vi "cs-scanning_v4.vi"() -> ()   [LabVIEW 2017]
uses:
  controls/boolean_info.ctl
  controls/TF-params.ctl
  controls/z-axis-params_v4.ctl
  <vilib>/rvi/Emulation/niFpgaGetClockAttributes.vi
  <vilib>/rvi/Emulation/niFpgaSctlEmulationGetInTimedLoop.vi
  <vilib>/rvi/Emulation/niFpgaEmulationReportErrorSimple.vi
  <vilib>/rvi/Emulation/niFpgaProcessEmulError.vi
  <vilib>/rvi/eio/common/nirviEmuTemplateMethod_errors.vi
  <vilib>/rvi/Emulation/niFpgaEmulationIsFPGAContextNoSignature.vi
  <vilib>/rvi/DataTransferAndStorage/Container/Common/niFpgaContainerGetUniqueNameForEmu.vi
  <vilib>/rvi/Memory/Memory_Emulation/niFpgaMemoryEmulationCacheClearOnFirstRun.vi
  <vilib>/rvi/Memory/Memory_Emulation/nirvimemoryEmulationManagerCache_MakeExclusive.vi
  <vilib>/rvi/Memory/Memory_Emulation/niFpgaMemoryEmulationValidateCache.vi
  <vilib>/rvi/Memory/Memory_Emulation/nirvimemoryEmulationManagerCache_InsertValue.vi
  <vilib>/Utility/error.llb/Clear Errors.vi
  <vilib>/rvi/Memory/Memory_Emulation/nirvimemoryEmulationManagerCache_ReleaseExclusive.vi
  <vilib>/rvi/Memory/Memory_Emulation/nirvimemoryEmulationManagerCache_GetValue.vi
  <vilib>/rvi/Memory/Memory_Emulation/nirvimemoryEmulationManagerCache_SetValue.vi
  <vilib>/rvi/Emulation/niFpgaCriticalErrorInLSC.vi
  <vilib>/eio/EIONode/EIONode.xnode
  <vilib>/rvi/DataTransferAndStorage/Container/XNode/niFpgaContainer.xnode
  <vilib>/rvi/DataTransferAndStorage/Register/Emulation/niFpgaRegisterEmulation.vi
  FPGA-data-logging.lvlib
  libimaging-cs.lvlib
panel:
  in  "z_axis_params":T1={"TOL"=0.3, "z_u_max"=5.0, "setpoint-scan"=0.0, "Ki-scan"=0.001, "Z_error_threshold"=0.0, "Z_settled_samples_threshold "=0, "uz_safe"=0.0, "Kiz_down"=0.001, "max_Z_settle_samples"=5000, "setpoint-up"=0.0} {"uz_safe" format="%#_13g"; "Z_error_threshold" format="%#_13g"; "TOL" format="%#_13g"}
  in  "TF-params":T2={"TF-order"=0, "Num"=[0.0, 0.0, 0.0, 0.0, 0.0, 0.0, 0.0, 0.0, 0.0], "Den"=[0.0, 0.0, 0.0, 0.0, 0.0, 0.0, 0.0, 0.0, 0.0]}
  in  "do-Dz":bool
  out "stop_loops":bool
  out "xy_k":fxp<+/-,16,5>[](array[numeric])
  out "xy_ref":fxp<+/-,16,5>[](array[numeric])
  out "u_x saturated":bool
  out "u_y saturated":bool
  out "state1-count":u64
  out "state5-count":u64
  out "state4-count":u64
  out "state3-count":u64
  out "state2-count":u64
  in  "collect all":bool
  out "entity-index":i16
  in  "TsTicks":u32=1600
  out "number-settled-samples-Z":i16
  out "Current Case":u8
  out "boolean \nindicators":T3
  out "z-u(k)":sgl
  in  "ABORT":bool
  out "read fifo timeout":bool
  in  "numEntities":i16
  in  "trigger-0":bool
  out "number-settled-samples-y":i16
  out "number-settled-samples-x":i16
  in  "xy-error-threshold":sgl format="%#_13g"
  in  "settled-samples\nthreshold":i16
  in  "Ki-xy":sgl=0.001 format="%#_13g"
  in  "xy-bound":sgl
  # "- If collect all = fasle ,\nwe only collect measurement data.\n- If collect all = true, we collect everything."
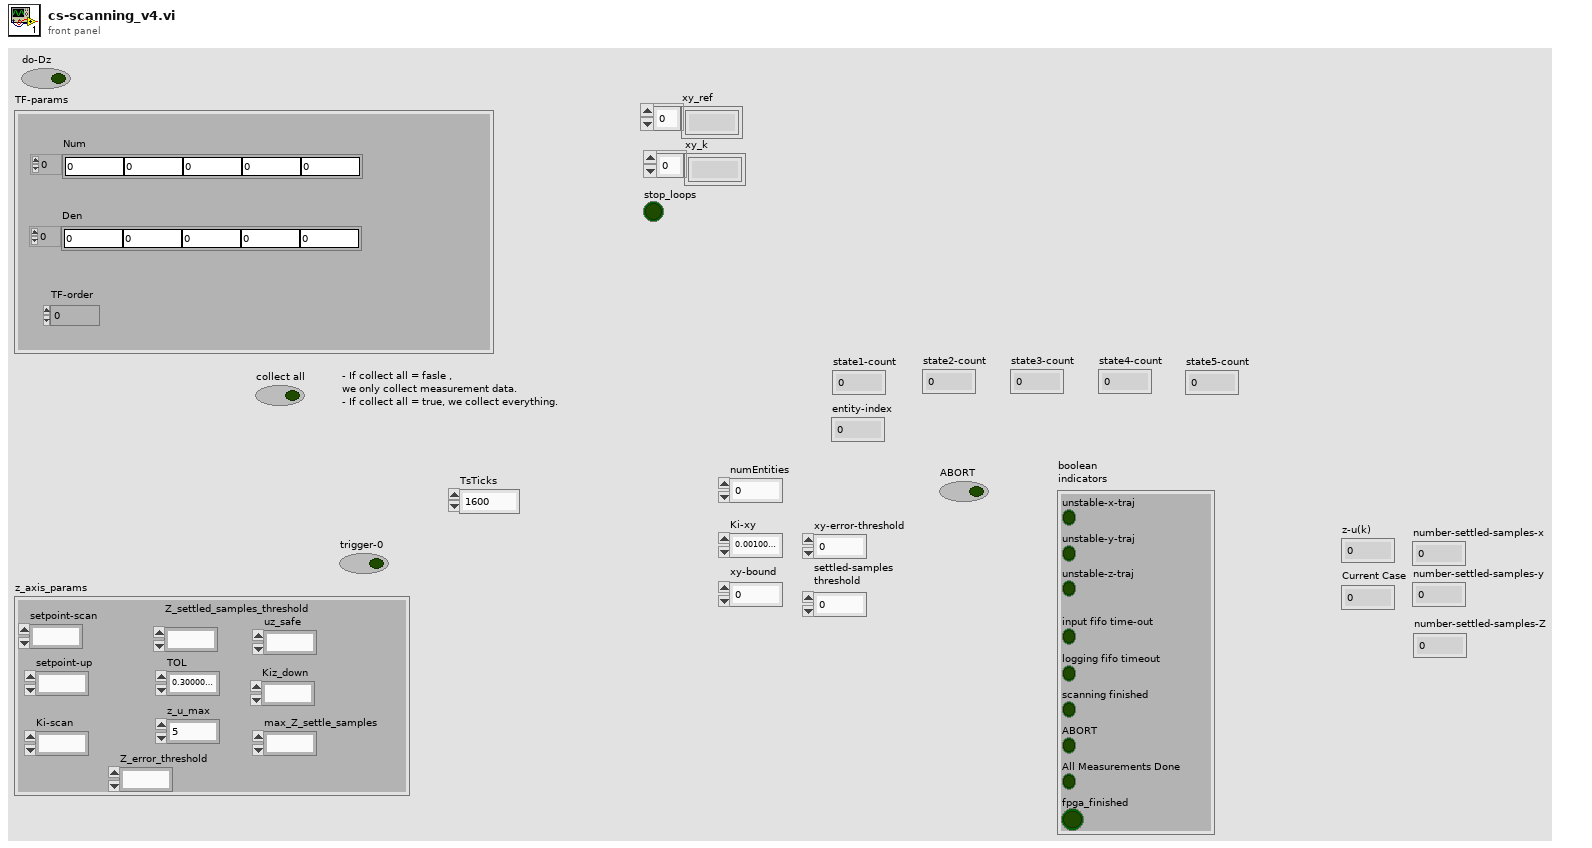
[diagram p1: front panel]
types:
  T1 = typedef "z-axis-params_v4.ctl" = cluster{"TOL":sgl, "z_u_max":sgl, "setpoint-scan":fxp<+/-,32,16>, "Ki-scan":sgl, "Z_error_threshold":sgl, "Z_settled_samples_threshold ":i16, "uz_safe":fxp<+/-,16,5>, "Kiz_down":sgl, "max_Z_settle_samples":i16, "setpoint-up":fxp<+/-,32,16>}
  T2 = typedef "TF-params.ctl" = cluster{"TF-order":i16, "Num":sgl[], "Den":sgl[]}
  T3 = typedef "boolean_info.ctl" = cluster{"unstable-z-traj":bool, "input fifo time-out":bool, "logging fifo timeout":bool, "scanning finished":bool, "unstable-x-traj":bool, "unstable-y-traj":bool, "ABORT":bool, "All Measurements Done":bool, "fpga_finished":bool}
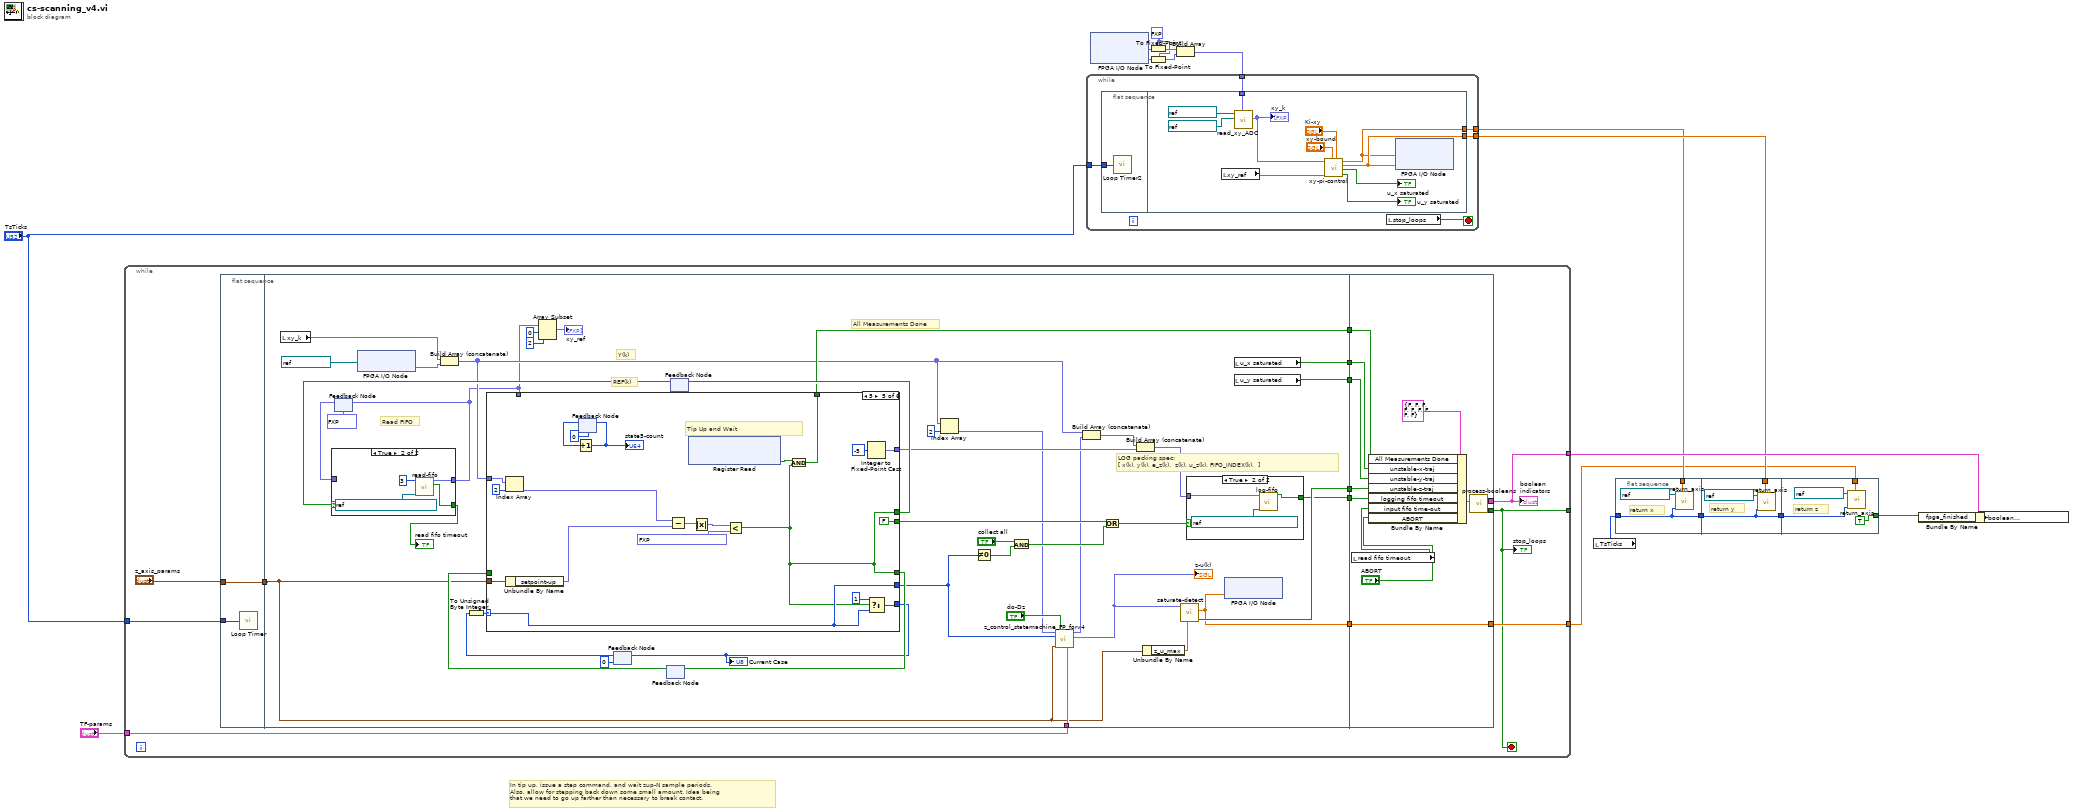
[diagram p0: block diagram]
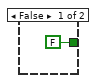
[diagram p2: hidden frame]
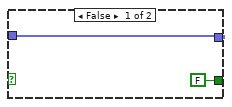
[diagram p3: hidden frame]
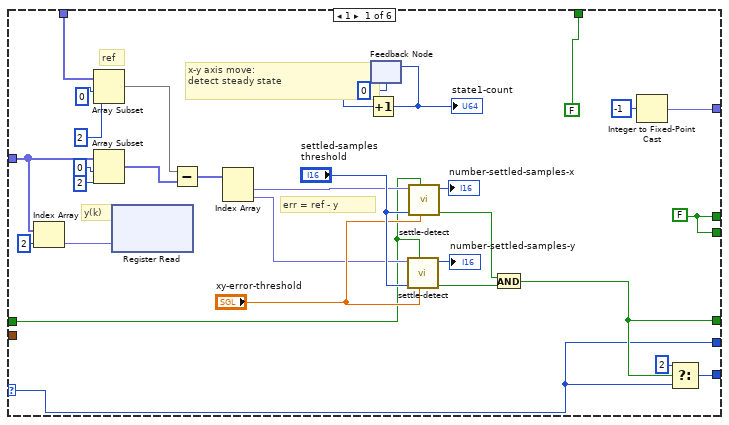
[diagram p4: hidden frame]
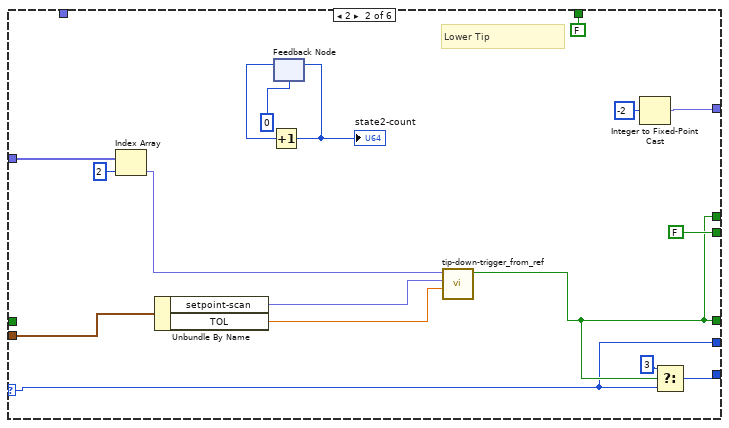
[diagram p5: hidden frame]
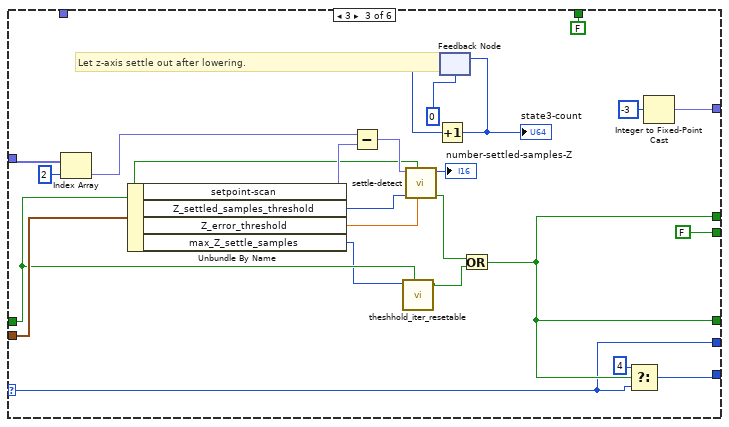
[diagram p6: hidden frame]
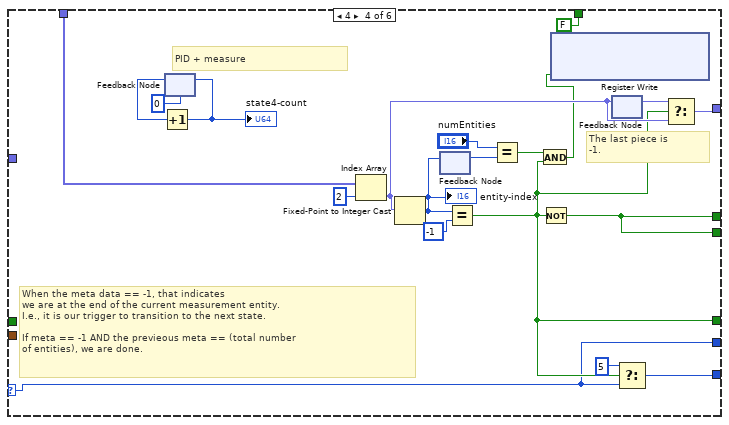
[diagram p7: hidden frame]
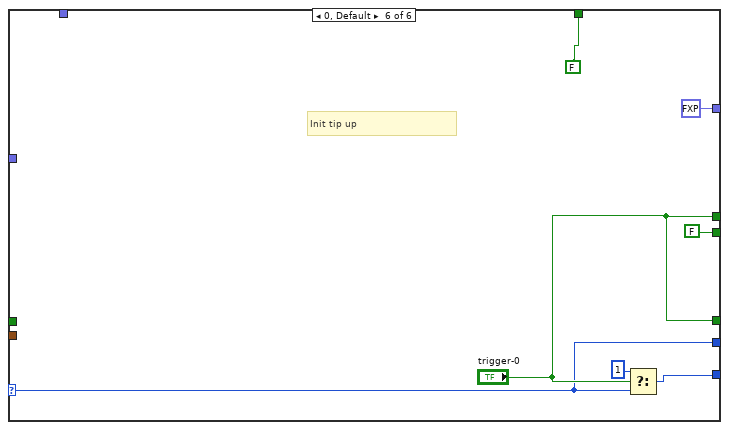
[diagram p8: hidden frame]
diagram:
  w13 = fxp<+/-,16,5> 0.0 ("fixed-point type")
  # "In tip up, issue a step command, and wait zup-N sample periods.\nAlso, allow for stepping back down some small amount. Idea being \nthat we need to go up farther than necessary to break contact."
  n1 = while {
    tunnel: "TsTicks" -> [w26]
    tunnel: [w22] -> _
    tunnel: [w24] -> w2
    tunnel: [w23] -> w9
    tunnel: "TF-params" -> [w19]
    stop <- w22 stop-if-true
    n2 = flat-sequence {
      tunnel: w26 -> [w31]
      tunnel: "z_axis_params" -> [w32]
      tunnel: [w32] -> w30
      tunnel: w30 -> [w33]
      tunnel: [w72] -> w29
      tunnel: [w71] -> w28
      tunnel: [w59] -> w27
      tunnel: [w40] -> w25
      tunnel: [w54] -> w21
      tunnel: [w53] -> w20
      tunnel: w19 -> [w38]
      tunnel: w29 -> [w215]
      tunnel: w28 -> [w212]
      tunnel: w27 -> [w209]
      tunnel: [w208] -> w22
      tunnel: [w207] -> w23
      tunnel: [w206] -> w24
      tunnel: w25 -> [w206]
      tunnel: w21 -> [w205]
      tunnel: w20 -> [w204]
      frame #0 {
        n3 = call "Loop Timer"("Count(Ticks)"=w31) -> ()  [unwired: 1 out]
      }
      frame #1 {
        # "All Measurements Done"
        # "REF(k)"
        # "Y(k)"
        # "LOG packing spec:\n[ x(k), y(k), e_z(k),  z(k), u_z(k), FIFO_INDEX(k),  ]"
        # "Read FIFO"
        n4 = local read "xy_k"() -> (w46:fxp<+/-,16,5>[])
        n5 = feedback #1(fxp<+/-,16,5>[] [0.0, 0.0, 0.0] ("unpacked-data")) -> (w74:fxp<+/-,16,5>[])
        n6 = xnode "FPGA I/O Node"("FPGA I/O In"=refnum<k21> "Mod2/AI2" ("y - ADC")) -> ("I/O Item"=w50:fxp<+/-,24,5>)  [unwired: 1 out]
        n7 = Build Array (concatenate)(w46, w50) -> (w49:fxp<+/-,24,5>[])
        n8 = feedback #2(u8 0 ("t")) -> (w44:u8)
        n9 = To Unsigned Byte Integer(number=w44) -> (unsigned 8bit integer=w45:u8)
        n10 = feedback #3() -> (w65:bool)  [unwired: 1 in]
        n11 = feedback #4() -> (w68:bool)  [unwired: 1 in]
        n12 = case shown="True" w68 {
          tunnel: w74 -> [w80 _]
          tunnel: [w80 w82] -> w41
          tunnel: [FALSE ("timout?") w81] -> w70
          frame False {
          }
          frame True {
            n13 = call "read-fifo.vi"("FIFO In"=refnum<k21> "host-to-fpga-fxp-16-5", "numChan"=3) -> ("timout?"=w81:bool, "unpacked-data"=w82:fxp<+/-,16,5>[])  [unwired: 8 in]
          }
        }
        "read fifo timeout" <- w70
        n14 = feedback-in #1(w41) -> ()
        n15 = case shown="5" w45 {
          selector: w45 -> [w85 w116 w134 w157 w184 w197]
          tunnel: [w86 FALSE FALSE ("trigger-0") w167 FALSE FALSE] -> w60
          tunnel: [w108 w128 w150 w175 w195 w203] -> w43
          tunnel: w49 -> [w87 w130 w154 _ w186 _]
          tunnel: [w86 w118 w137 w167 w179 "trigger-0"] -> w69
          tunnel: w33 -> [_ w132 w148 _ w178 _]
          tunnel: [FALSE FALSE FALSE FALSE w188 FALSE] -> w59
          tunnel: w41 -> [w99 _ _ w169 _ _]
          tunnel: w65 -> [w97 _ w135 _ _ _]
          tunnel: [w96 w118 w137 w160 w179 "trigger-0"] -> w66
          tunnel: [w90 w119 w140 w163 w189 fxp<+/-,16,5> 0.0 ("Element")] -> w47
          tunnel: [w85 w116 w134 w157 w184 w197] -> w36
          frame 1 {
            w86 = FALSE
            # "y(k)"
            # "err = ref - y"
            # "ref"
            # "x-y axis move: \ndetect steady state"
            n16 = Index Array(array=w87, index=2) -> (element=w89:fxp<+/-,24,5>)
            n17 = Array Subset(array=w99, index=0, length=2) -> (w103:fxp<+/-,16,5>[])
            n18 = Array Subset(array=w87, index=0, length=2) -> (w102:fxp<+/-,24,5>[])
            n19 = xnode ("Register Read")("Data"=w89) -> ()  [unwired: 1 in, 1 out]
            n20 = Subtract(x=w103, y=w102) -> (x-y=w95:fxp<+/-,25,6>[])
            n21 = Index Array(array=w95) -> (element #1=w101:fxp<+/-,25,6>, element #2=w100:fxp<+/-,25,6>)  [unwired: 2 in]
            n22 = feedback #5(u64 0) -> (w93:u64)
            n23 = Increment(x=w93) -> (x+1=w94:u64)
            "state1-count" <- w94
            n24 = feedback-in #5(w94) -> ()
            n25 = call "settle-detect.vi"("error-max"="xy-error-threshold", "reset"=w97, "settled-samples\nthreshold"="settled-samples\nthreshold", "err(k)"=w100) -> ("has-settled"=w115:bool, "number-settled-samples"=→"number-settled-samples-y":u16)  [unwired: 6 in]
            n26 = call "settle-detect.vi"("error-max"="xy-error-threshold", "reset"=w97, "settled-samples\nthreshold"="settled-samples\nthreshold", "err(k)"=w101) -> ("has-settled"=w114:bool, "number-settled-samples"=→"number-settled-samples-x":u16)  [unwired: 6 in]
            n27 = And(x=w114, y=w115) -> (x .and. y?=w96:bool)
            n28 = Integer to Fixed-Point Cast(integer=i16 -1) -> (fixed-point=w90:fxp<+/-,16,5>)  [unwired: 1 in]
            n29 = Select(t=u8 2, s=w96, f=w85) -> (s? t:f=w108:u8)
          }
          frame 2 {
            # "Lower Tip"
            n30 = Index Array(array=w130, index=2) -> (element=w129:fxp<+/-,24,5>)
            n31 = Unbundle By Name(w132) -> ("setpoint-scan"=w120:fxp<+/-,32,16>, "TOL"=w117:sgl)
            n32 = feedback #6(u64 0) -> (w123:u64)
            n33 = Increment(x=w123) -> (x+1=w124:u64)
            "state2-count" <- w124
            n34 = feedback-in #6(w124) -> ()
            n35 = call "tip-down-trigger_from_ref.vi"("TOL"=w117, "setpoint"=w120, "I/O Item"=w129) -> ("Boolean"=w118:bool)  [unwired: 8 in]
            n36 = Integer to Fixed-Point Cast(integer=i16 -2) -> (fixed-point=w119:fxp<+/-,16,5>)  [unwired: 1 in]
            n37 = Select(t=u8 3, s=w118, f=w116) -> (s? t:f=w128:u8)
          }
          frame 3 {
            # "Let z-axis settle out after lowering."
            n38 = Index Array(array=w154, index=2) -> (element=w152:fxp<+/-,24,5>)
            n39 = Unbundle By Name(w148) -> ("setpoint-scan"=w139:fxp<+/-,32,16>, "Z_settled_samples_threshold"=w147:i16, "Z_error_threshold"=w146:sgl, "max_Z_settle_samples"=w133:i16)
            n40 = Subtract(x=w152, y=w139) -> (x-y=w155:fxp<+/-,36,17>)
            n41 = call "theshhold_iter_resetable.vi"("reset"=w135, "N"=w133) -> ("Boolean"=w136:bool)  [unwired: 8 in, 1 out]
            n42 = call "settle-detect.vi"("error-max"=w146, "reset"=w135, "settled-samples\nthreshold"=w147, "err(k)"=w155) -> ("has-settled"=w138:bool, "number-settled-samples"=→"number-settled-samples-Z":u16)  [unwired: 6 in]
            n43 = feedback #7(u64 0) -> (w143:u64)
            n44 = Increment(x=w143) -> (x+1=w144:u64)
            "state3-count" <- w144
            n45 = feedback-in #7(w144) -> ()
            n46 = Or(x=w138, y=w136) -> (x .or. y?=w137:bool)
            n47 = Select(t=u8 4, s=w137, f=w134) -> (s? t:f=w150:u8)
            n48 = Integer to Fixed-Point Cast(integer=i16 -3) -> (fixed-point=w140:fxp<+/-,16,5>)  [unwired: 1 in]
          }
          frame 4 {
            # "The last piece is\n-1."
            # "When the meta data == -1, that indicates\nwe are at the end of the current measurement entity.\nI.e., it is our trigger to transition to the next state.\n\nIf meta == -1 AND the previeous meta == (total number\nof entities), we are done."
            # "PID + measure"
            n49 = feedback #8(u64 0) -> (w165:u64)
            n50 = Increment(x=w165) -> (x+1=w166:u64)
            "state4-count" <- w166
            n51 = feedback-in #8(w166) -> ()
            n52 = Index Array(array=w169, index=2) -> (element=w161:fxp<+/-,16,5>)
            n53 = Fixed-Point to Integer Cast(1:w161) -> (0:w168:i16)
            "entity-index" <- w168
            n54 = feedback #9() -> (w170:i16)  [unwired: 1 in]
            n55 = feedback-in #9(w168) -> ()
            n56 = Equal?(x=w168, y=i16 -1) -> (x = y?=w160:bool)
            n57 = Equal?(x="numEntities", y=w170) -> (x = y?=w171:bool)
            n58 = And(x=w171, y=w160) -> (x .and. y?=w159:bool)
            n59 = Not(x=w160) -> (.not. x?=w167:bool)
            n60 = xnode ("Register Write")("Data"=w159) -> ()  [unwired: 1 in, 1 out]
            n61 = feedback #10() -> (w162:fxp<+/-,16,5>)  [unwired: 1 in]
            n62 = feedback-in #10(w161) -> ()
            n63 = Select(t=u8 5, s=w160, f=w157) -> (s? t:f=w175:u8)
            n64 = Select(t=w162, s=w160, f=w161) -> (s? t:f=w163:fxp<+/-,16,5>)
          }
          frame 5 {
            # "Tip Up and Wait"
            n65 = Index Array(array=w186, index=2) -> (element=w183:fxp<+/-,24,5>)
            n66 = Unbundle By Name(w178) -> ("setpoint-up"=w177:fxp<+/-,32,16>)
            n67 = feedback #11(u64 0) -> (w192:u64)
            n68 = Increment(x=w192) -> (x+1=w193:u64)
            "state5-count" <- w193
            n69 = feedback-in #11(w193) -> ()
            n70 = Subtract(x=w183, y=w177) -> (x-y=w182:fxp<+/-,36,17>)
            n71 = xnode ("Register Read")() -> ("Data"=w185:bool)  [unwired: 1 in, 1 out]
            n72 = Absolute Value(x=w182) -> (abs(x)=w181:fxp<+,35,16>)
            n73 = Less?(x=w181, y=fxp<+,24,5> 0.10000038146972656) -> (x < y?=w179:bool)
            n74 = And(x=w185, y=w179) -> (x .and. y?=w188:bool)
            n75 = Integer to Fixed-Point Cast(integer=i16 -5) -> (fixed-point=w189:fxp<+/-,16,5>)  [unwired: 1 in]
            n76 = Select(t=u8 1, s=w179, f=w184) -> (s? t:f=w195:u8)
          }
          frame 0, Default {
            # "Init tip up"
            n77 = Select(t=u8 1, s="trigger-0", f=w197) -> (s? t:f=w203:u8)
          }
        }
        "Current Case" <- w43
        n78 = Array Subset(array=w41, index=0, length=2) -> (→"xy_ref":fxp<+/-,16,5>[])
        n79 = feedback-in #2(w43) -> ()
        n80 = feedback-in #3(w66) -> ()
        n81 = feedback-in #4(w69) -> ()
        n82 = Index Array(array=w49, index=2) -> (element=w35:fxp<+/-,24,5>)
        n83 = Not Equal To 0?(x=w36) -> (x != 0?=w63:bool)
        n84 = And(x="collect all", y=w63) -> (x .and. y?=w61:bool)
        n85 = call "z_control_statemachine_FP_forv4.vi"("TF-params"=w38, "do-Dz"="do-Dz", "z_axis_params"=w33, "State"=w36, "zerr(k)"=w35) -> ("zuk_Dinv"=w39:fxp<+/-,16,5>, "z-u(k)"=w34:fxp<+/-,16,5>)  [unwired: 5 in]
        "z-u(k)" <- w39
        n86 = Build Array (concatenate)(w49, w34) -> (w48:fxp<+/-,24,5>[])
        n87 = Or(x=w60, y=w61) -> (x .or. y?=w64:bool)
        n88 = Build Array (concatenate)(w48, w47) -> (w73:fxp<+/-,24,5>[])
        n89 = Unbundle By Name(w33) -> ("z_u_max"=w57:sgl)
        n90 = call "saturate-detect.vi"("bound"=w57, "x"=w39) -> ("saturated"=w72:bool, "sat(x)"=w40:sgl)  [unwired: 8 in]
        n91 = case shown="True" w64 {
          tunnel: w73 -> [_ w77]
          tunnel: [FALSE ("logging-timeout?") w76] -> w71
          frame False {
          }
          frame True {
            n92 = call "log-fifo.vi"("FIFO In"=refnum<k21> "fpga-to-host2-fxp-16-5", "input-data"=w77) -> ("logging-timeout?"=w76:bool)  [unwired: 9 in]
          }
        }
        n93 = xnode "FPGA I/O Node"("Mod1/AO2"=w40) -> ()  [unwired: 1 in, 1 out]
        n94 = local read "u_x saturated"() -> (w54:bool)
        n95 = local read "u_y saturated"() -> (w53:bool)
      }
      frame #2 {
        n96 = local read "read fifo timeout"() -> (w211:bool)
        n97 = Bundle By Name(cluster=T3 {"unstable-z-traj"=FALSE, "input fifo time-out"=FALSE, "logging fifo timeout"=FALSE, "scanning finished"=FALSE, "unstable-x-traj"=FALSE, "unstable-y-traj"=FALSE, "ABORT"=FALSE, "All Measurements Done"=FALSE, "fpga_finished"=FALSE} ("boolean errors"), "All Measurements Done"=w209, "unstable-x-traj"=w205, "unstable-y-traj"=w204, "unstable-z-traj"=w215, "logging fifo timeout"=w212, "input fifo time-out"=w211, "ABORT"="ABORT") -> (w213:T3)
        n98 = call "process-booleans.vi"("boolean indicators 2"=w213) -> ("scaning finished"=w208:bool, "boolean indicators"=w207:T3)  [unwired: 9 in]
      }
    }
    "boolean \nindicators" <- w23
    "stop_loops" <- w22
  }
  n99 = xnode "FPGA I/O Node"() -> ("Mod2/AI0"=w16:fxp<+/-,24,5>, "Mod2/AI1"=w14:fxp<+/-,24,5>)  [unwired: 2 in, 2 out]
  n100 = To Fixed-Point(fixed-point type=w13, number=w16) -> (fixed-point=w17:fxp<+/-,16,5>)
  n101 = To Fixed-Point(fixed-point type=w13, number=w14) -> (fixed-point=w15:fxp<+/-,16,5>)
  n102 = Build Array(w17, w15) -> (w3:fxp<+/-,16,5>[])
  n103 = while {
    tunnel: "TsTicks" -> [w220]
    tunnel: [w219] -> w5
    tunnel: [w218] -> w4
    tunnel: w3 -> [w217]
    stop <- w216 stop-if-true
    n104 = flat-sequence {
      tunnel: w220 -> [w221]
      tunnel: [w231] -> w219
      tunnel: [w230] -> w218
      tunnel: w217 -> [w226]
      frame #0 {
        n105 = call "Loop Timer2"("Count(Ticks)"=w221) -> ()  [unwired: 1 out]
      }
      frame #1 {
        n106 = local read "xy_ref"() -> (w223:fxp<+/-,16,5>[])
        n107 = call "read_xy_ADC.vi"("x(0), y(0)"=w226, "y - ADC"=refnum<k21> "Mod2/AI1", "x - ADC"=refnum<k21> "Mod2/AI0") -> ("x_y"=w222:fxp<+/-,17,6>[])  [unwired: 8 in]
        "xy_k" <- w222
        n108 = call "xy-pi-control.vi"("Ki-xy"="Ki-xy", "xy-umax"="xy-bound", "xy-ref"=w223, "x_k-y_k"=w222) -> ("u_y saturated"=→"u_y saturated":bool, "u_x saturated"=→"u_x saturated":bool, "sat(u_y)"=w231:sgl, "sat(u_x)"=w230:sgl)  [unwired: 4 in]
        n109 = xnode "FPGA I/O Node"("Mod1/AO0"=w230, "Mod1/AO1"=w231) -> ()  [unwired: 2 in, 2 out]
      }
    }
    n110 = local read "stop_loops"() -> (w216:bool)
  }
  n111 = local read "TsTicks"() -> (w10:u32)
  n112 = flat-sequence {
    tunnel: w10 -> [w234]
    tunnel: w4 -> [w235]
    tunnel: [w234] -> w12
    tunnel: w5 -> [w238]
    tunnel: w12 -> [w236]
    tunnel: [w236] -> w11
    tunnel: w2 -> [w242]
    tunnel: w11 -> [w240]
    tunnel: [TRUE] -> w8
    frame #0 {
      # "return x"
      n113 = call "return_axis.vi"("u(0)"=w235, "TsTicks"=w234, "FPGA I/O In"=refnum<k21> "Mod1/AO0") -> ()  [unwired: 9 in]
    }
    frame #1 {
      # "return y"
      n114 = call "return_axis.vi"("u(0)"=w238, "TsTicks"=w236, "FPGA I/O In"=refnum<k21> "Mod1/AO1") -> ()  [unwired: 9 in]
    }
    frame #2 {
      # "return z"
      n115 = call "return_axis.vi"("u(0)"=w242, "TsTicks"=w240, "FPGA I/O In"=refnum<k21> "Mod1/AO2") -> ()  [unwired: 9 in]
    }
  }
  n116 = Bundle By Name(cluster=w9, "fpga_finished"=w8) -> (w7:T3)
  n117 = local write "boolean \nindicators"(w7) -> ()
